vi "Programa de labview DAQ SIN WAIT.vi"() -> ()   [LabVIEW 2014]
uses:
  <vilib>/Instr/_visa.llb/Select Event Type.ctl
panel:
  out "return count":u32
  out "ENTRADAS PUERTO D":bool[](array[boolean])
  out "Thermometer":dbl(slide) scale=0.0..255.0
  out "CONT":dbl
  out "AN6":dbl
  out "AN5":dbl
  out "AN4":dbl
  out "AN3":dbl
  out "AN2":dbl
  out "AN1":dbl
  in  "PWM 1":u8(slide)=30 scale=0.0..255.0
  in  "PWM 2":u8(slide)=41 scale=0.0..255.0
  in  "SALIDAS PUERTO B":bool[](array[boolean])
  out "Byte enviado":u32
  in  "stop":bool
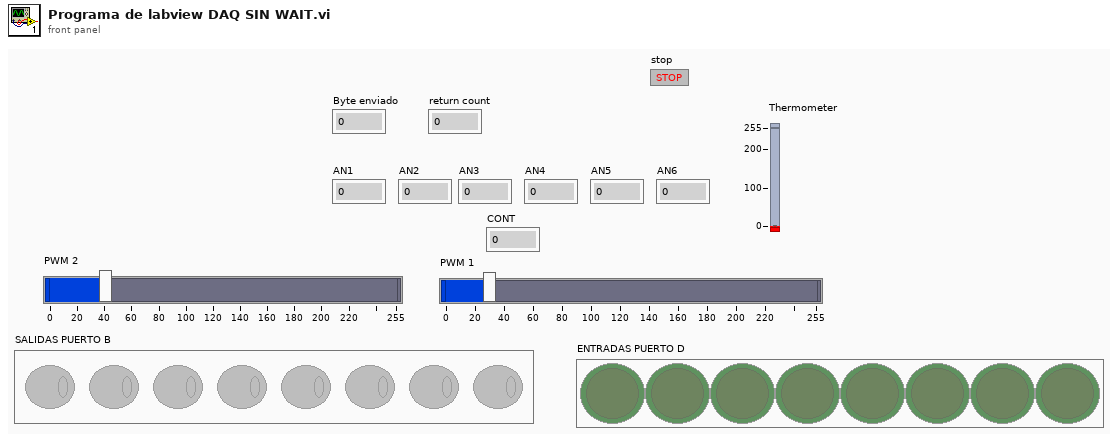
[diagram p1: front panel]
types:
  T1 = typedef "Select Event Type.ctl" = u32
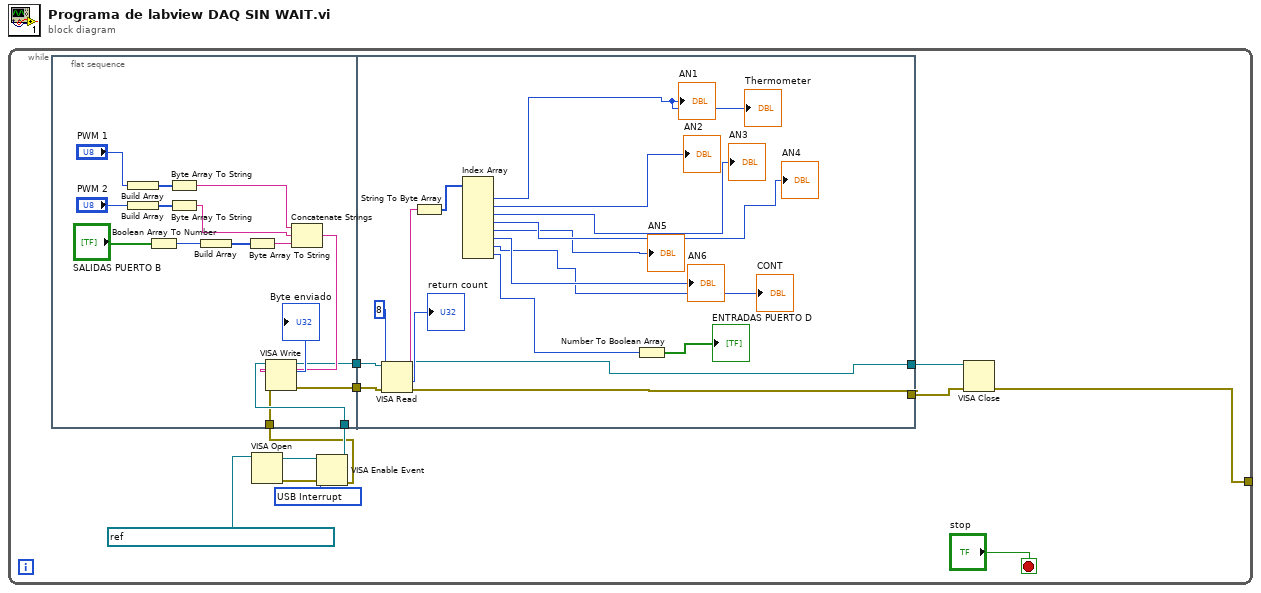
[diagram p0: block diagram]
diagram:
  n1 = while {
    tunnel: [w11] -> _
    stop <- "stop" stop-if-true
    w8 = T1 1073684535 items=["Service Request"=1073684491, "Trigger"=3221168138, "Clear"=1073684493, "VXI Signal"=1073684512, "VXI/VME Interrupt"=3221168161, "VXI/VME Sysfail"=1073684509, "VXI/VME Sysreset"=1073684510, "GPIB CIC"=1073684498, "GPIB Talk"=1073684499, "GPIB Listen"=1073684500, "PXI Interrupt"=1073684514, "Serial Break"=1073684515, "Serial TermChar"=1073684516, "Serial CTS"=1073684521, "Serial DSR"=1073684522, "Serial DCD"=1073684524, "Serial RI"=1073684526, "Serial Character"=1073684533, "USB Interrupt"=1073684535, "All Enabled"=1073709055] ("Event Type")
    n2 = flat-sequence {
      tunnel: w6 -> [w16]
      tunnel: w5 -> [w15]
      tunnel: [w14] -> w4
      tunnel: [w13] -> w3
      tunnel: w4 -> [w32]
      tunnel: w3 -> [w31]
      tunnel: [w30] -> w2
      tunnel: [w29] -> w1
      frame #0 {
        n3 = Build Array("PWM 1") -> (w22:u8[])
        n4 = Build Array("PWM 2") -> (w20:u8[])
        n5 = Boolean Array To Number(Boolean array="SALIDAS PUERTO B") -> (number=w26:u32)
        n6 = Byte Array To String(unsigned byte array=w22) -> (string=w18:string)
        n7 = Byte Array To String(unsigned byte array=w20) -> (string=w19:string)
        n8 = Build Array(w26) -> (w27:u32[])
        n9 = Byte Array To String(unsigned byte array=w27) -> (string=w25:string)
        n10 = Concatenate Strings(w18, w19, w25) -> (w17:string)
        n11 = VISA Write(VISA resource name=w16, write buffer=w17, error in (no error)=w15) -> (VISA resource name out=w14:refnum<visa-resource-name>, return count=→"Byte enviado":u32, error out=w13:errorcluster)
      }
      frame #1 {
        n12 = VISA Read(VISA resource name=w32, byte count=u32 8 ("General Settings:Timeout Value"), error in (no error)=w31) -> (VISA resource name out=w30:refnum<visa-resource-name>, read buffer=w43:string, return count=→"return count":u32, error out=w29:errorcluster)
        n13 = String To Byte Array(string=w43) -> (unsigned byte array=w41:u8[])
        n14 = Index Array(array=w41) -> (element #1=→"AN1" →"Thermometer":u8, element #2=→"AN2":u8, element #3=→"AN3":u8, element #4=→"AN4":u8, element #5=→"AN5":u8, element #6=→"AN6":u8, element #7=→"CONT":u8, element #8=w33:u8)  [unwired: 8 in]
        n15 = Number To Boolean Array(number=w33) -> (Boolean array=→"ENTRADAS PUERTO D":bool[])
      }
    }
    n16 = VISA Open(VISA resource name=refnum<visa-resource-name> "USB0::0x0461::0x0020::NI-VISA-0::RAW") -> (VISA resource name=w10:refnum<visa-resource-name>, error out=w9:errorcluster)  [unwired: 4 in]
    n17 = VISA Enable Event(8:w9, 10:w8, 11:w10) -> (0:w5:errorcluster, 3:w6:refnum<visa-resource-name>)  [unwired: 1 in]
    n18 = VISA Close(VISA resource name=w2, error in (no error)=w1) -> (error out=w11:errorcluster)
  }
